vi "Write InstrumentCommunication.vi"(8 "error in (no error)":errorcluster, 10 "InstrumentCommunication":string[][](array[string]), 11 "UnitTestEngine in":refnum<class "UnitTestEngine.lvclass">) -> (0 "error out":errorcluster, 3 "UnitTestEngine out":refnum<class "UnitTestEngine.lvclass">)   [LabVIEW 2019, in "UnitTestEngine.lvlib" / "UnitTestEngine.lvclass"]
uses:
  UnitTestEngine.lvclass
  UnitTestEngine.lvclass/UnitTestEngine.ctl
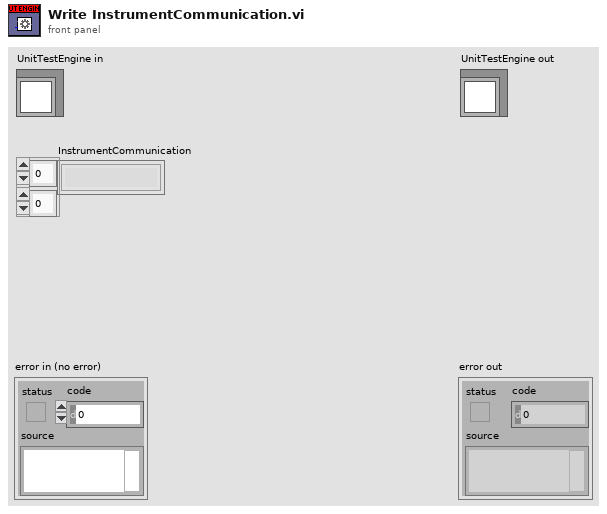
[diagram p1: front panel]
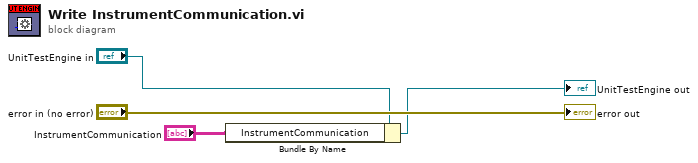
[diagram p0: block diagram]
diagram:
  n1 = Bundle By Name(cluster="UnitTestEngine in", "InstrumentCommunication"="InstrumentCommunication") -> (→"UnitTestEngine out":refnum<class "UnitTestEngine.lvclass">)
  "error out" <- "error in (no error)"
